vi "Write State.vi"(8 "error in (no error)":errorcluster, 10 "State":refnum<class "State Pattern.lvclass">, 11 "A Context State in":refnum<class "A Context State.lvclass">) -> (0 "error out":errorcluster, 3 "A Context State out":refnum<class "A Context State.lvclass">)   [LabVIEW 2021, in "A Context State.lvclass"]
uses:
  State Pattern/State Pattern.lvclass
  A Context State.lvclass
  A Context State.lvclass/A Context State.ctl
  Context/Context.lvclass
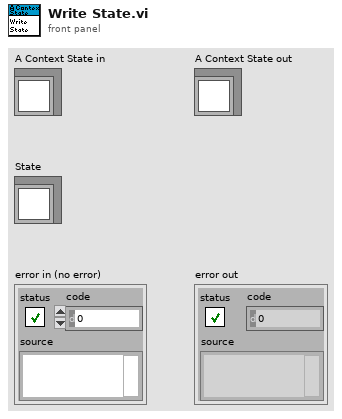
[diagram p1: front panel]
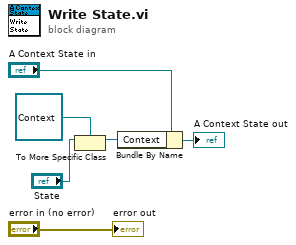
[diagram p0: block diagram]
diagram:
  n1 = To More Specific Class(target class=refnum<class "Context.lvclass"> refnum ("Context.lvclass"), reference="State") -> (specific class reference=w3:refnum<class "Context.lvclass">)  [unwired: 1 in, 1 out]
  n2 = Bundle By Name(cluster="A Context State in", "Context"=w3) -> (→"A Context State out":refnum<class "A Context State.lvclass">)
  "error out" <- "error in (no error)"
